vi "SDG60ConfSTDWFM.vi"(1 "Frequency/Period (1 Hz/s)":dbl=2.0 format="%#.16g", 2 "DC Offset (0.00 V)":dbl format="%#_15g", 5 "Channel (1:Channel 1)":i32(ring)=1 items=["Channel 1"=1, "Channel 2"=2], 7 "Waveform Function (0: Sine)":u16(ring) items=["Sine", "Square", "Ramp", "DC", "Pulse", "Arb"], 9 "Amplitude (1.0 Vpp)":dbl=0.1 format="%#.6f", 11 "Phase (0.0 degrees)":dbl min=-360.0 max=360.0 format="%#.15g", 12 "Symmetry/Duty (50.0 %)":dbl=50.0 format="%#.6f") -> ()   [LabVIEW 2022 SP3]
doc: "Selects the waveform shape, frequency, amplitude, offset, and phase for standard waveforms (including Sine, Square, Ramp, Pulse, DC and Arb).\n\nNotes: \nTo configure other parameters for pulse waveforms please run the Configure Pulse VI. \nTo configure noise waveform please run the Configure Noise VI.\nTo configure other parameters for arbitrary waveforms please run the Create Arbitrary Waveform. \nTo configure PRBS waveform please run the Configure PRBS Waveform VI."
uses:
  <vilib>/addons/zeromq/socket_type.ctl
  <vilib>/addons/zeromq/zmq_context.lvclass
  <vilib>/addons/zeromq/zmq_socket.lvclass
  <vilib>/addons/zeromq/zeromq.lvlib
panel:
  out "Python response":string
  out "error out":errorcluster
  # "For Noise use seperate vi\nFor ARB, must follow up with SDG60ConfArbWaveform.\nIf using user ARB, precede with SDG60CreateArbWaveform.\nFor pulse must follow up with seperate vi to change parameters (in fact don't need this vi to set pulses at all)"
  # "0.1mV resolution"
  # "Range: 1 uHz-200 MHz  (Sine)\nRange: 20 ns-1 Ms\nInternal setting max res 10 digits for freq, 6 digits for period"
  # "Ignored for all but Ramp and Square\nSymmetry range :0%-100%\nDuty range: 0.001%-Max depends on freq\n6 digit precision (~73..99%)"
  # "0.1mV resolution"
  # "Res: 0.001 degree. Range +/-279 deg"
  # "Operating sequence in case output is already on:\nWhen run, will turn off output for ~150ms\nthen turn use set waveform\nthen freq change\nthen amp change\nthen use DC offset\nthen use phase offset (discontiouse)"
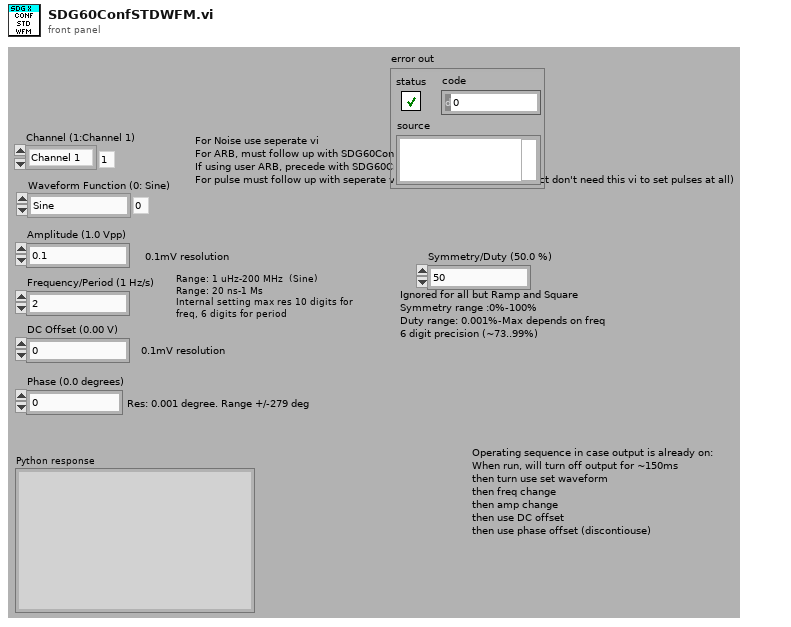
[diagram p1: front panel]
types:
  T1 = typedef "zeromq.lvlib/socket_type.ctl" = enum8{"ZMQ_PAIR", "ZMQ_PUB", "ZMQ_SUB", "ZMQ_REQ", "ZMQ_REP", "ZMQ_DEALER", "ZMQ_ROUTER", "ZMQ_PULL", "ZMQ_PUSH", "ZMQ_XPUB", "ZMQ_XSUB", "ZMQ_STREAM", "ZMQ_SERVER", "ZMQ_CLIENT", "ZMQ_RADIO", "ZMQ_DISH", "ZMQ_GATHER", "ZMQ_SCATTER", "ZMQ_DGRAM"}
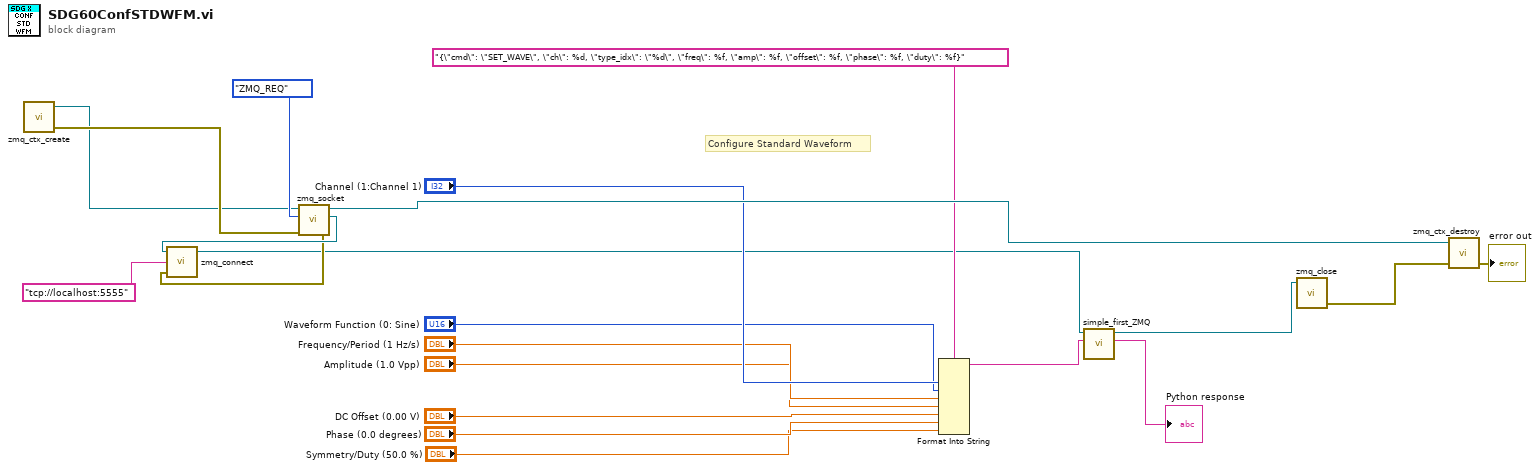
[diagram p0: block diagram]
diagram:
  # "Configure Standard Waveform"
  n1 = call <vilib>:"zmq_ctx_create.vi"() -> ("error out"=w16:errorcluster, "context out"=w13:refnum<class "zmq_context.lvclass">)  [unwired: 4 in]
  n2 = call <vilib>:"zmq_socket.vi"("error in"=w16, "socket type"=socket_type."ZMQ_REQ", "context in"=w13) -> ("error out"=w15:errorcluster, "socket out"=w20:refnum<class "zmq_socket.lvclass">, "context out"=w19:refnum<class "zmq_context.lvclass">)  [unwired: 2 in]
  n3 = call <vilib>:"zmq_connect.vi"("error in"=w15, "endpoint"="tcp://localhost:5555", "socket in"=w20) -> ("socket out"=w4:refnum<class "zmq_socket.lvclass">)  [unwired: 1 in, 1 out]
  n4 = Format Into String(format string="{\"cmd\": \"SET_WAVE\", \"ch\": %d, \"type_idx\": \"%d\", \"freq\": %f, \"amp\": %f, \"offset\": %f, \"phase\": %f, \"duty\": %f}", "Channel (1:Channel 1)", "Waveform Function (0: Sine)", "Frequency/Period (1 Hz/s)", "Amplitude (1.0 Vpp)", "DC Offset (0.00 V)", "Phase (0.0 degrees)", "Symmetry/Duty (50.0 %)") -> (resulting string=w5:string)  [unwired: 2 in, 1 out]
  n5 = call "simple_first_ZMQ.vi"("Raw command"=w5, "ZMQ socket in"=w4) -> ("Python response"=→"Python response":string, "ZMQ socket out"=w3:refnum<class "zmq_socket.lvclass">)  [unwired: 4 in]
  n6 = call <vilib>:"zmq_close.vi"("socket"=w3) -> ("error out"=w18:errorcluster)  [unwired: 4 in]
  n7 = call <vilib>:"zmq_ctx_destroy.vi"("error in"=w18, "context in"=w19) -> ("error out"=→"error out":errorcluster)  [unwired: 3 in]
